vi "itemNames.vi"(9 "pair":i32, 10 "StatusRef":refnum<vi>, 11 "itemName":string) -> (2 "itemNameArray":string[](array[string]))   [LabVIEW 2011]
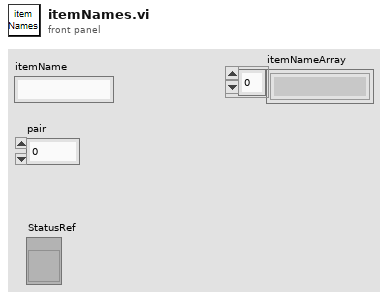
[diagram p1: front panel]
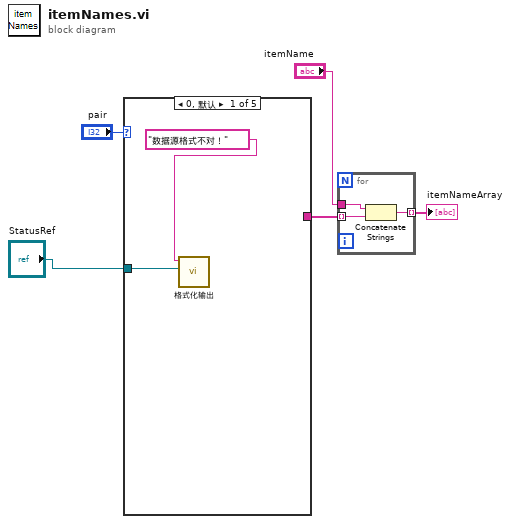
[diagram p0: block diagram]
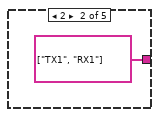
[diagram p2: hidden frame]
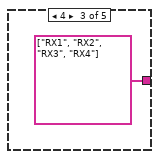
[diagram p3: hidden frame]
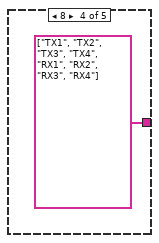
[diagram p4: hidden frame]
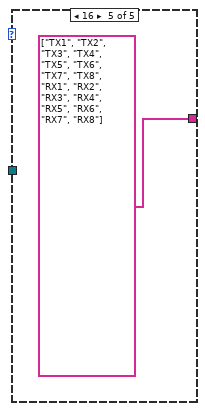
[diagram p5: hidden frame]
diagram:
  n1 = case shown="0, 默认" "pair" {
    tunnel: [_ string[] ["TX1", "RX1"] string[] ["RX1", "RX2", "RX3", "RX4"] string[] ["TX1", "TX2", "TX3", "TX4", "RX1", "RX2", "RX3", "RX4"] string[] ["TX1", "TX2", "TX3", "TX4", "TX5", "TX6", "TX7", "TX8", "RX1", "RX2", "RX3", "RX4", "RX5", "RX6", "RX7", "RX8"]] -> w4
    tunnel: "StatusRef" -> [w6 _ _ _ _]
    frame 0, Default {
      n2 = call "格式化输出.vi"("字符串引用"=w6, "字符串"="数据源格式不对！" ("消息")) -> ()  [unwired: 9 in, 1 out]
    }
    frame 2 {
    }
    frame 4 {
    }
    frame 8 {
    }
    frame 16 {
    }
  }
  n3 = for {
    tunnel: w4 -> [w14] mode=indexing
    tunnel: "itemName" -> [w13]
    tunnel: [w12] -> w2 mode=indexing
    n4 = Concatenate Strings(w13, w14) -> (w12:string)
  }
  "itemNameArray" <- w2
